vi "Async Handler.vi"(8 "error in (no error)":errorcluster, 9 "Message Data":variant, 10 "Message":string, 11 "Asynchronous Action In":refnum<class "Async Handler.lvclass">) -> (0 "error out":errorcluster, 3 "Asynchronous Action Out":refnum<class "Async Handler.lvclass">)   [LabVIEW 2020, in "Async Handler.lvclass"]
uses:
  Async Handler.lvclass
  Error Handler Interface/Error Handler Interface.lvclass
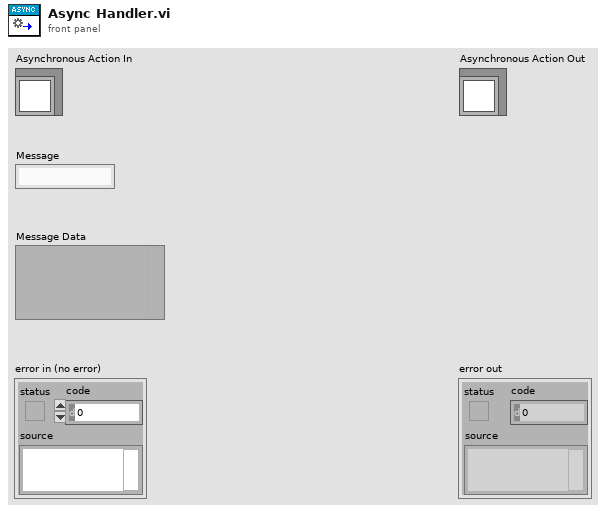
[diagram p1: front panel]
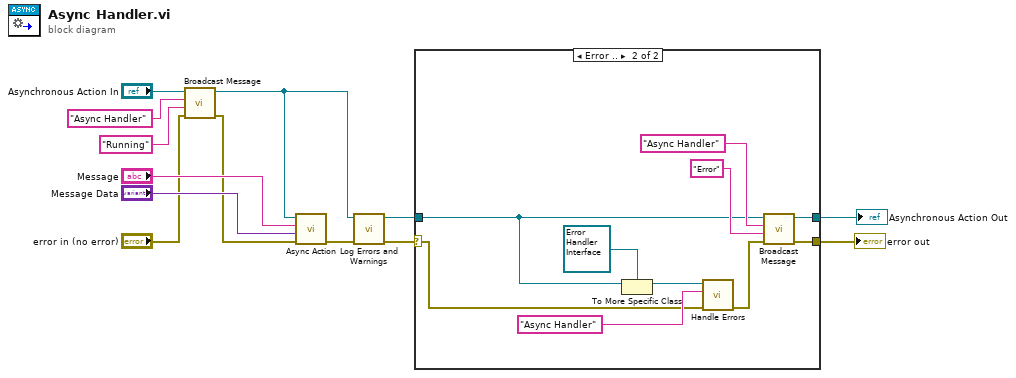
[diagram p0: block diagram]
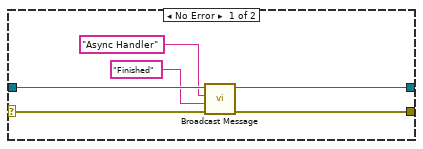
[diagram p2: hidden frame]
diagram:
  n1 = call-dynamic "Broadcast Message.vi"("error in (no error)"="error in (no error)", "Message Data"="Running" ("Message"), "Message"="Async Handler", "Asynchronous Action In"="Asynchronous Action In") -> ("error out"=w7:errorcluster, "Asynchronous Action Out"=w2:refnum<class "Async Handler.lvclass">)  [unwired: 6 in]
  n2 = call-dynamic "Async Action.vi"("error in (no error)"=w7, "Message Data"="Message Data", "Message"="Message", "Async Handler In"=w2) -> ("error out"=w4:errorcluster)  [unwired: 7 in]
  n3 = call "Log Errors and Warnings.vi"("error in (no error)"=w4, "Async Handler in"=w2) -> ("error out"=w3:errorcluster, "Async Handler out"=w1:refnum<class "Async Handler.lvclass">)  [unwired: 8 in]
  n4 = case shown="Error .." w3 {
    selector: w3 -> [w17 w20]
    tunnel: w1 -> [w18 w21]
    tunnel: [w19 w27] -> w11
    tunnel: [w16 w25] -> w10
    frame No Error {
      n5 = call-dynamic "Broadcast Message.vi"("error in (no error)"=w17, "Message Data"="Finished" ("Message"), "Message"="Async Handler", "Asynchronous Action In"=w18) -> ("error out"=w16:errorcluster, "Asynchronous Action Out"=w19:refnum<class "Async Handler.lvclass">)  [unwired: 6 in]
    }
    frame Error {
      n6 = To More Specific Class(target class=refnum<class "Error Handler Interface.lvclass"> refnum ("Process In"), reference=w21) -> (specific class reference=w22:refnum<class "Error Handler Interface.lvclass">)  [unwired: 1 in, 1 out]
      n7 = call-dynamic "Handle Errors.vi"("error in (no error)"=w20, "Location"="Async Handler" ("format string"), "Error Handler Interface In"=w22) -> ("error out"=w26:errorcluster)  [unwired: 7 in, 1 out]
      n8 = call-dynamic "Broadcast Message.vi"("error in (no error)"=w26, "Message Data"="Error" ("Message"), "Message"="Async Handler", "Asynchronous Action In"=w21) -> ("error out"=w25:errorcluster, "Asynchronous Action Out"=w27:refnum<class "Async Handler.lvclass">)  [unwired: 6 in]
    }
  }
  "error out" <- w10
  "Asynchronous Action Out" <- w11
